vi "Teardown.vi"(8 "Error In":errorcluster, 11 "Lexer":refnum<class "Lexer.lvclass">) -> (0 "Error Out":errorcluster)   [LabVIEW 2018, in "Tests.lvlib" / "Lexer.lvlib"]
uses:
  Lexer.lvlib
  src/Toolkit/Low-Level/Lexer/Lexer.lvclass
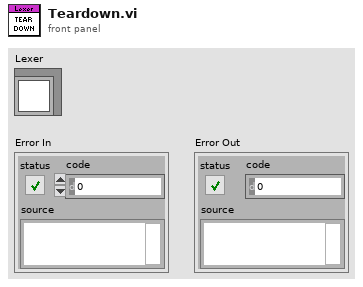
[diagram p1: front panel]
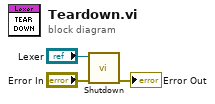
[diagram p0: block diagram]
diagram:
  n1 = call-dynamic "Shutdown.vi"("Error In"="Error In", "Lexer In"="Lexer") -> ("Error Out"=→"Error Out":errorcluster)  [unwired: 8 in, 1 out]
